vi "GlobalAutonomous.vi"() -> ()   [LabVIEW 2023]
doc: "These global variables report autonomous sequencing and path following data."
panel:
  out "Auto_Shooter_Prespin":bool
  out "Auto_Reverse_Intake":bool
  out "Legal_Auto_Plays":string[](array[string])
  out "Auto_Sequence_Complete":bool
  out "Auto_Rumble_Driver_Joystick":bool
  out "Auto_Path_Suffix":string
  out "Auto_Error":errorcluster
  out "Distance_From_Start (in)":dbl
  out "Distance_From_End (in)":dbl
  out "Auto_Manipulator_Step":i32
  out "Auto_Drive_Step":i32
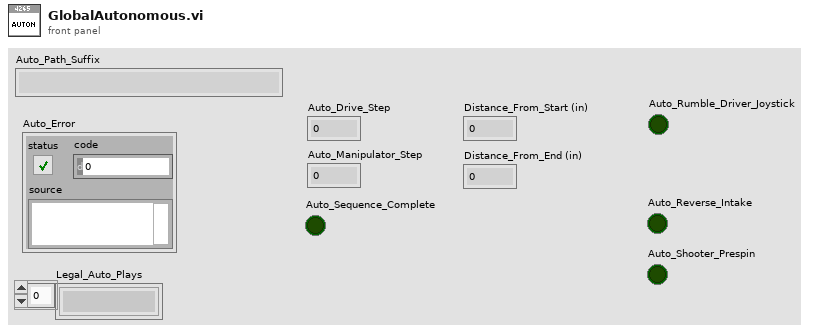
[diagram p1: front panel]
diagram:
